vi "Main.vi"() -> ()   [LabVIEW 2019]
uses:
  Moveo.lvclass
  MoveoSerialClass/MoveoSerial.lvclass
panel:
  in  "Speed Wrist":i16(slide)=303 scale=0.0..1000.0
  in  "Speed Elbow":i16(slide)=303 scale=0.0..1500.0
  in  "Speed Shoulder":i16(slide)=51 scale=0.0..800.0
  out "Recive":string
  in  "Move Wrist":bool
  in  "Wrist":dbl
  in  "Elbow":dbl
  in  "Move Elbow":bool
  in  "Shoulder":dbl
  in  "Move Shoulder":bool
  in  "Disable Motors":bool
  in  "Enable Motors":bool
  in  "Rotary Arm":dbl
  in  "Move Rotary Arm":bool
  in  "Base":dbl
  in  "MoveBase":bool
  in  "VISA resource name":refnum<visa-resource-name>
  in  "Stopp":bool
  in  "Close Gripper":bool
  in  "Open Gripper":bool
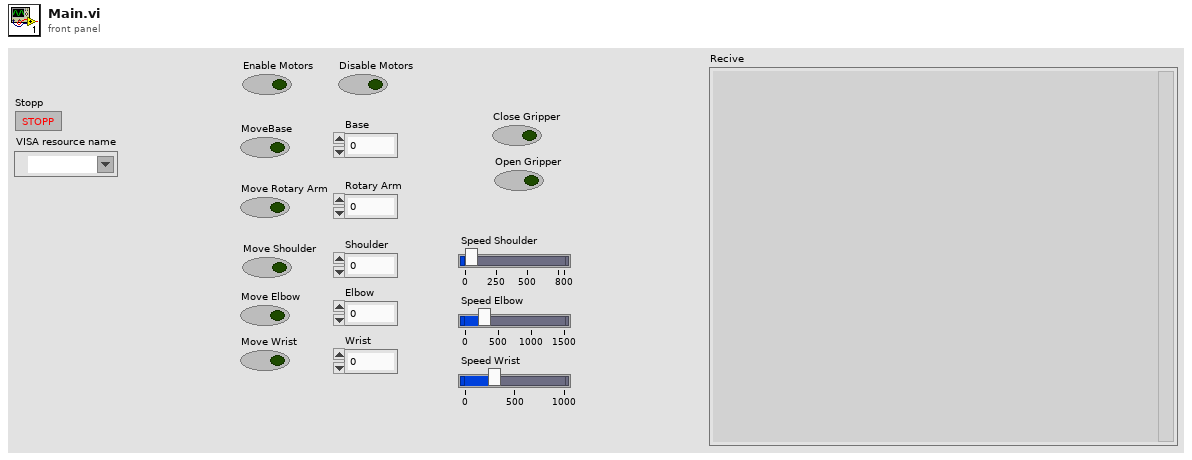
[diagram p1: front panel]
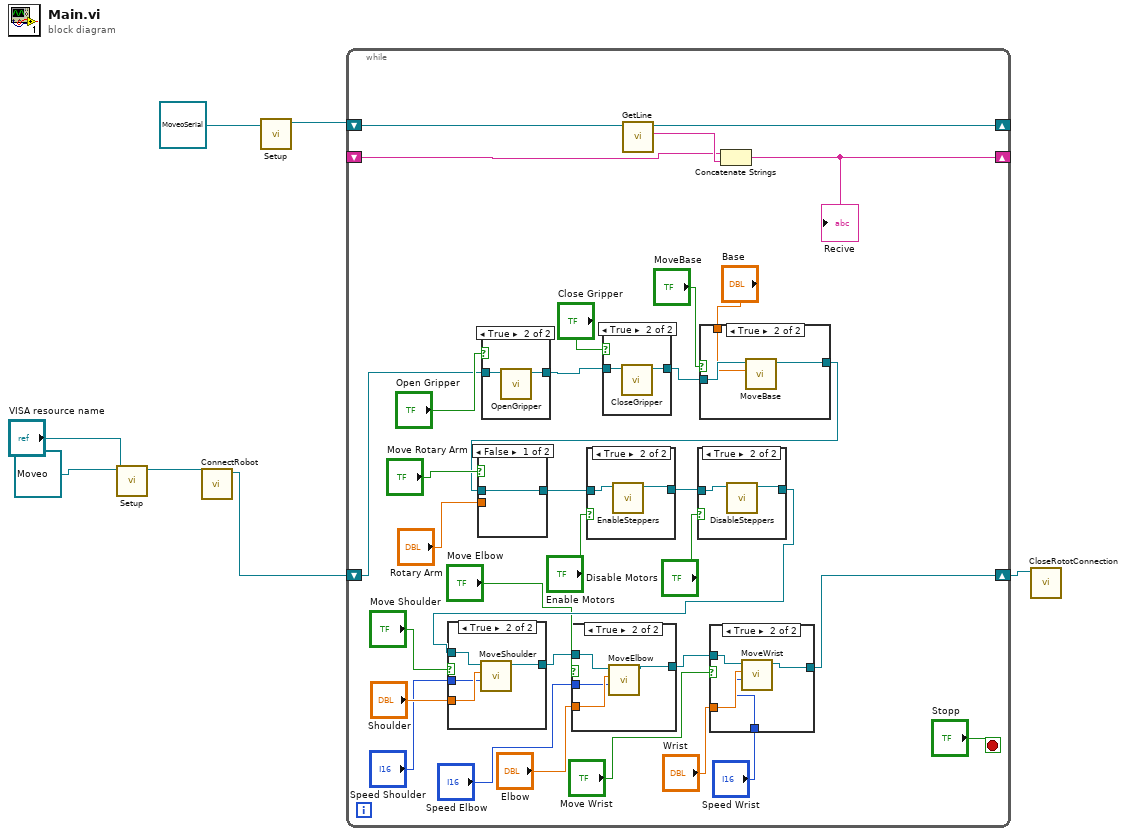
[diagram p0: block diagram]
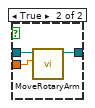
[diagram p7: hidden frame]
diagram:
  n1 = call-dynamic "Setup.vi"("VISA resource name"="VISA resource name", "Moveo Eingang"=refnum<class "Moveo.lvclass"> refnum ("Moveo.lvclass")) -> ("Moveo Ausgang"=w6:refnum<class "Moveo.lvclass">)  [unwired: 8 in, 1 out]
  n2 = call-dynamic "ConnectRobot.vi"("Moveo Eingang"=w6) -> ("Moveo Ausgang"=w5:refnum<class "Moveo.lvclass">)  [unwired: 9 in, 1 out]
  n3 = call-dynamic "Setup.vi"("MoveoSerial Eingang"=refnum<class "MoveoSerial.lvclass"> refnum ("MoveoSerial.lvclass")) -> ("MoveoSerial Ausgang"=w1:refnum<class "MoveoSerial.lvclass">)  [unwired: 9 in, 1 out]
  n4 = while {
    shift-right: [w17] -> w4
    shift-left: w5 -> [w38]
    shift-right: [w14] -> _
    shift-left: w1 -> [w15]
    shift-right: [w12] -> _
    shift-left: _ -> [w11]
    stop <- "Stopp" stop-if-true
    n5 = case shown="True" "Open Gripper" {
      tunnel: w38 -> [w73 w75]
      tunnel: [w73 w74] -> w37
      frame False {
      }
      frame True {
        n6 = call-dynamic "OpenGripper.vi"("Moveo Eingang"=w75) -> ("Moveo Ausgang"=w74:refnum<class "Moveo.lvclass">)  [unwired: 9 in, 1 out]
      }
    }
    n7 = case shown="True" "Close Gripper" {
      tunnel: w37 -> [w70 w72]
      tunnel: [w70 w71] -> w34
      frame False {
      }
      frame True {
        n8 = call-dynamic "CloseGripper.vi"("Moveo Eingang"=w72) -> ("Moveo Ausgang"=w71:refnum<class "Moveo.lvclass">)  [unwired: 9 in, 1 out]
      }
    }
    n9 = call-dynamic "GetLine.vi"("MoveoSerial Eingang"=w15) -> ("RecivedLine"=w13:string, "MoveoSerial Ausgang"=w14:refnum<class "MoveoSerial.lvclass">)  [unwired: 8 in, 1 out]
    n10 = case shown="True" "MoveBase" {
      tunnel: w34 -> [w66 w69]
      tunnel: "Base" -> [_ w68]
      tunnel: [w66 w67] -> w31
      frame False {
      }
      frame True {
        n11 = call-dynamic "MoveBase.vi"("Base"=w68, "Moveo Eingang"=w69) -> ("Moveo Ausgang"=w67:refnum<class "Moveo.lvclass">)  [unwired: 8 in, 1 out]
      }
    }
    n12 = case shown="False" "Move Rotary Arm" {
      tunnel: w31 -> [w62 w65]
      tunnel: "Rotary Arm" -> [_ w64]
      tunnel: [w62 w63] -> w29
      frame False {
      }
      frame True {
        n13 = call-dynamic "MoveRotaryArm.vi"("Rotary Arm"=w64, "Moveo Eingang"=w65) -> ("Moveo Ausgang"=w63:refnum<class "Moveo.lvclass">)  [unwired: 8 in, 1 out]
      }
    }
    n14 = case shown="True" "Enable Motors" {
      tunnel: w29 -> [w59 w61]
      tunnel: [w59 w60] -> w28
      frame False {
      }
      frame True {
        n15 = call-dynamic "EnableSteppers.vi"("Moveo Eingang"=w61) -> ("Moveo Ausgang"=w60:refnum<class "Moveo.lvclass">)  [unwired: 9 in, 1 out]
      }
    }
    n16 = case shown="True" "Disable Motors" {
      tunnel: w28 -> [w56 w58]
      tunnel: [w56 w57] -> w24
      frame False {
      }
      frame True {
        n17 = call-dynamic "DisableSteppers.vi"("Moveo Eingang"=w58) -> ("Moveo Ausgang"=w57:refnum<class "Moveo.lvclass">)  [unwired: 9 in, 1 out]
      }
    }
    n18 = case shown="True" "Move Shoulder" {
      tunnel: w24 -> [w51 w55]
      tunnel: "Shoulder" -> [_ w54]
      tunnel: [w51 w53] -> w22
      tunnel: "Speed Shoulder" -> [_ w52]
      frame False {
      }
      frame True {
        n19 = call-dynamic "MoveShoulder.vi"("Speed"=w52, "Shoulder"=w54, "Moveo Eingang"=w55) -> ("Moveo Ausgang"=w53:refnum<class "Moveo.lvclass">)  [unwired: 7 in, 1 out]
      }
    }
    n20 = case shown="True" "Move Elbow" {
      tunnel: w22 -> [w46 w50]
      tunnel: [w46 w48] -> w19
      tunnel: "Elbow" -> [_ w49]
      tunnel: "Speed Elbow" -> [_ w47]
      frame False {
      }
      frame True {
        n21 = call "MoveElbow.vi"("Speed"=w47, "Elbow"=w49, "Moveo Eingang"=w50) -> ("Moveo Ausgang"=w48:refnum<class "Moveo.lvclass">)  [unwired: 7 in, 1 out]
      }
    }
    n22 = case shown="True" "Move Wrist" {
      tunnel: w19 -> [w41 w45]
      tunnel: [w41 w43] -> w17
      tunnel: "Wrist" -> [_ w44]
      tunnel: "Speed Wrist" -> [_ w42]
      frame False {
      }
      frame True {
        n23 = call "MoveWrist.vi"("Speed"=w42, "Wrist"=w44, "Moveo Eingang"=w45) -> ("Moveo Ausgang"=w43:refnum<class "Moveo.lvclass">)  [unwired: 7 in, 1 out]
      }
    }
    n24 = Concatenate Strings(w11, w13) -> (w12:string)
    "Recive" <- w12
  }
  n25 = call-dynamic "CloseRototConnection.vi"("Moveo Eingang"=w4) -> ()  [unwired: 9 in, 2 out]
